vi "log.write.path.vi"(8 "error in":errorcluster, 10 "dataSourceRid":string) -> (0 "error out":errorcluster, 3 "path":string)   [LabVIEW 2020, in "Nominal Client.lvclass"]
uses:
  Nominal Client.lvclass
  Nominal Client.lvclass/Nominal Client.ctl
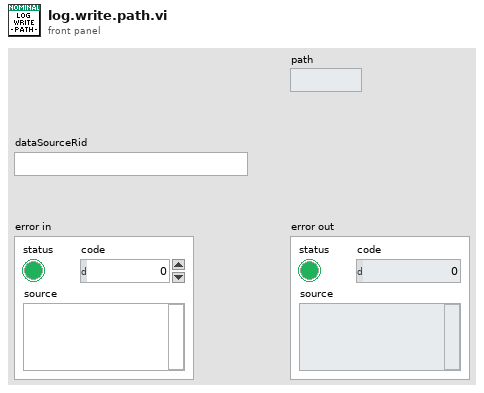
[diagram p1: front panel]
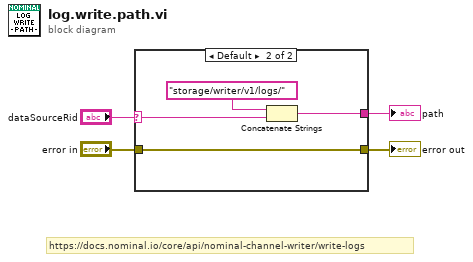
[diagram p0: block diagram]
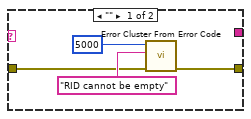
[diagram p2: hidden frame]
diagram:
  # "https://docs.nominal.io/core/api/nominal-channel-writer/write-logs"
  n1 = case shown="Default" "dataSourceRid" {
    selector: "dataSourceRid" -> [_ w12]
    tunnel: [_ w10] -> w3
    tunnel: "error in" -> [w6 w9]
    tunnel: [w5 w9] -> w1
    frame "" {
      n2 = call <vilib>:"Error Cluster From Error Code.vi"("error in (no error)"=w6, "error message (\"\")"="RID cannot be empty" ("error message (\"\")"), "error code (0)"=5000) -> ("error out"=w5:errorcluster)  [unwired: 6 in]
    }
    frame Default {
      n3 = Concatenate Strings("storage/writer/v1/logs/" ("Path"), w12) -> (w10:string)
    }
  }
  "error out" <- w1
  "path" <- w3
